vi "NXT_ Init Behavior Data.vi"() -> (0 "Behavior Data":T1)   [LabVIEW 2012, in "Tugboat.lvrbt"]
uses:
  Tugboat.lvrbt
  behaviorData_t.ctl
  behaviorOutput_t.ctl
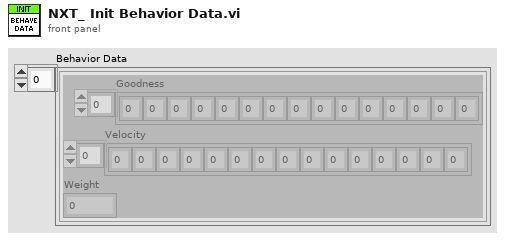
[diagram p1: front panel]
types:
  T1 = typedef "behaviorData_t.ctl" = T2[]
  T2 = typedef "behaviorOutput_t.ctl" = cluster{"Goodness":i8[], "Velocity":i8[], "Weight":i8}
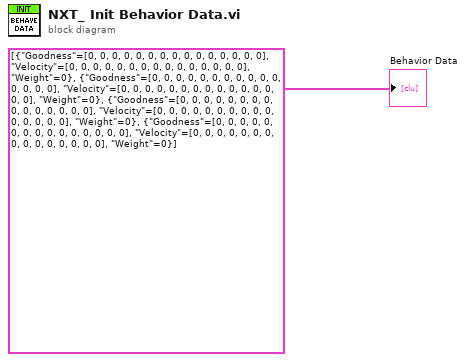
[diagram p0: block diagram]
diagram:
  "Behavior Data" <- T1 [{"Goodness"=[0, 0, 0, 0, 0, 0, 0, 0, 0, 0, 0, 0, 0, 0, 0], "Velocity"=[0, 0, 0, 0, 0, 0, 0, 0, 0, 0, 0, 0, 0, 0, 0], "Weight"=0}, {"Goodness"=[0, 0, 0, 0, 0, 0, 0, 0, 0, 0, 0, 0, 0, 0, 0], "Velocity"=[0, 0, 0, 0, 0, 0, 0, 0, 0, 0, 0, 0, 0, 0, 0], "Weight"=0}, {"Goodness"=[0, 0, 0, 0, 0, 0, 0, 0, 0, 0, 0, 0, 0, 0, 0], "Velocity"=[0, 0, 0, 0, 0, 0, 0, 0, 0, 0, 0, 0, 0, 0, 0], "Weight"=0}, {"Goodness"=[0, 0, 0, 0, 0, 0, 0, 0, 0, 0, 0, 0, 0, 0, 0], "Velocity"=[0, 0, 0, 0, 0, 0, 0, 0, 0, 0, 0, 0, 0, 0, 0], "Weight"=0}] ("Behavior Data")
